vi "Buffer Connections List_Actions.vi"(0 "Connection Cluster":T2, 1 "Connections Ref":T3, 2 "State":T1=enum."Update", 7 "index":i32, 11 "error in (no error)":errorcluster) -> (3 "Connections Ref out":T3, 4 "Connections":T2[](array[typedef]), 8 "Connection Cluster Out":T2, 15 "error out":errorcluster {"code" min=0 max=0})   [LabVIEW 2015, in "J1939 Addon Engine.lvlib"]
uses:
  Engine/J1939 Addon Engine.lvlib
  Types/BAM Buffer Connections List_Ref.ctl
  Types/TP Buffer Connection Cluster.ctl
  Types/TP Connections List State.ctl
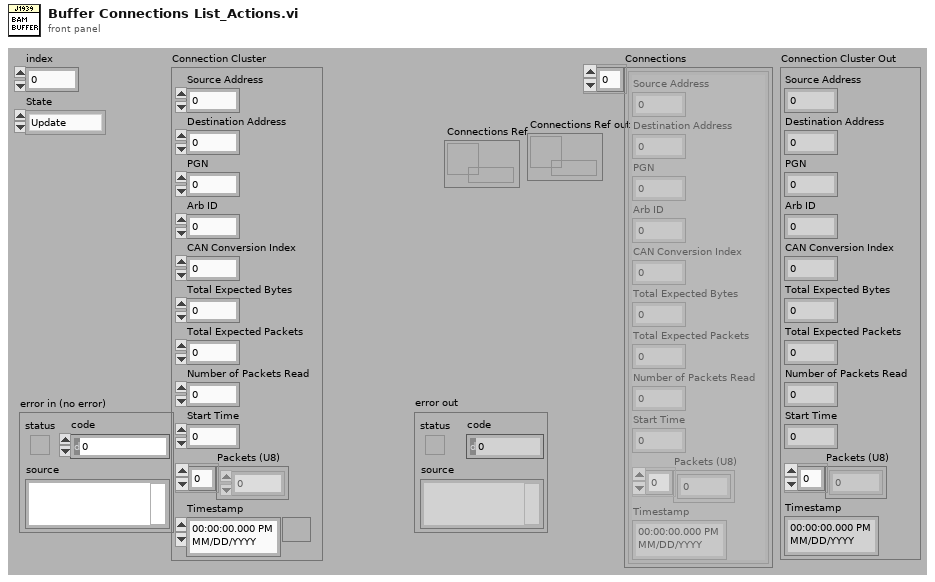
[diagram p1: front panel]
types:
  T1 = typedef "J1939 Addon Engine.lvlib/TP Connections List State.ctl" = enum16{"Add", "Update", "Get", "Remove", "Initialize"}
  T2 = typedef "J1939 Addon Engine.lvlib/TP Buffer Connection Cluster.ctl" = cluster{"Source Address":u8, "Destination Address":u8, "PGN":u32, "Arb ID":u32, "CAN Conversion Index":u32, "Total Expected Bytes":u16, "Total Expected Packets":u8, "Number of Packets Read":u8, "Start Time":u32, "Packets (U8)":u8[], "Timestamp":timestamp}
  T3 = typedef "J1939 Addon Engine.lvlib/BAM Buffer Connections List_Ref.ctl" = refnum<data-value>
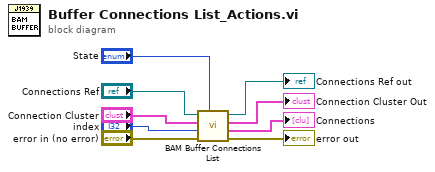
[diagram p0: block diagram]
diagram:
  n1 = call "BAM Buffer Connections List.vi"("State"="State", "error in (no error)"="error in (no error)", "index"="index", "Connection Cluster"="Connection Cluster", "Connections Ref"="Connections Ref") -> ("error out"=→"error out":errorcluster, "Connections"=→"Connections":T2[], "Connection Cluster Out"=→"Connection Cluster Out":T2, "Connections Ref out"=→"Connections Ref out":T3)  [unwired: 3 in]
